vi "GetNumberLevelsExpanded.vi"(8 "error in (no error)":errorcluster, 9 "ClassName Cache":refnum<data-value>, 10 "To object (more specific)":refnum<class>, 11 "From object (less specific)":refnum<class>) -> (0 "error out":errorcluster, 3 "NumLevelsExpanded":u32)   [LabVIEW 2020, in "BlueSerialization.lvlib" / "BlueSerializer.lvclass"]
uses:
  BlueSerializer.lvclass
  ClassNameCacheMap.ctl
  ClassNameObj.ctl
  Support/GetParentClassesHiererchy.vi
  ClassNameCacheWrite.vi
  LVOOP Get Default Object Inline.vi
  <vilib>/Utility/LVClass/Get LV Class Name.vi
  <vilib>/Utility/LVClass/Get LV Class Default Value By Name.vi
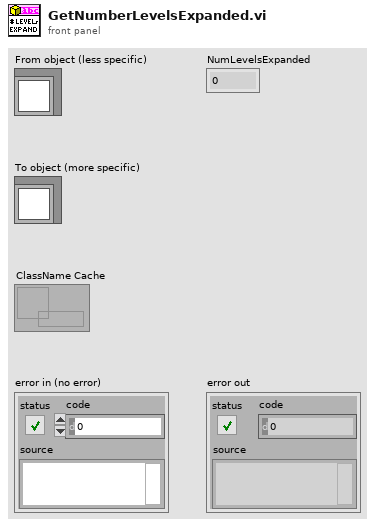
[diagram p1: front panel]
types:
  T1 = typedef "BlueSerialization.lvlib/BlueSerializer.lvclass/ClassNameObj.ctl" = cluster{"class name":string, "default object":refnum<class>}
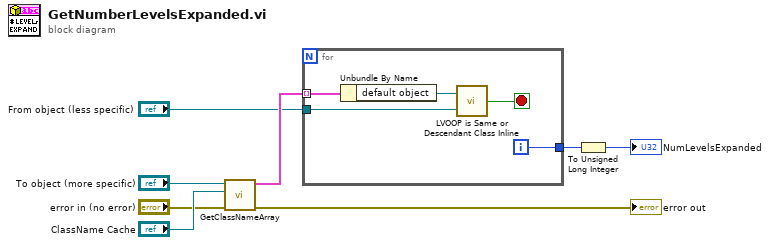
[diagram p0: block diagram]
diagram:
  n1 = call "GetClassNameArray.vi"("error in (no error)"="error in (no error)", "ClassName Cache"="ClassName Cache", "LabVIEW Object in"="To object (more specific)") -> ("error out"=→"error out":errorcluster, "Class (child,parent)"=w8:T1[])  [unwired: 7 in]
  n2 = for {
    tunnel: w8 -> [w13] mode=indexing
    tunnel: "From object (less specific)" -> [w10]
    tunnel: [w12] -> w2
    i -> [w12]
    stop <- w9 stop-if-true
    n3 = Unbundle By Name(w13) -> ("default object"=w11:refnum<class>)
    n4 = call "LVOOP is Same or Descendant Class Inline.vi"("Possible Descendant Object"=w10, "Object"=w11) -> ("Is Same Class or Descendant?"=w9:bool)
  }
  n5 = To Unsigned Long Integer(number=w2) -> (unsigned 32bit integer=→"NumLevelsExpanded":u32)
